vi "Read Peels.vi"(8 "error in (no error)":errorcluster, 11 "Banana in":refnum<class "Banana.lvclass">) -> (0 "error out":errorcluster, 2 "Peels":set{refnum<class "BananaPeel.lvclass">}(c389), 3 "Banana out":refnum<class "Banana.lvclass">)   [LabVIEW 2021, in "Bananas.lvlib" / "Banana.lvclass"]
uses:
  Banana.lvclass
  Banana.lvclass/Banana.ctl
  BananaPeel/BananaPeel.lvclass
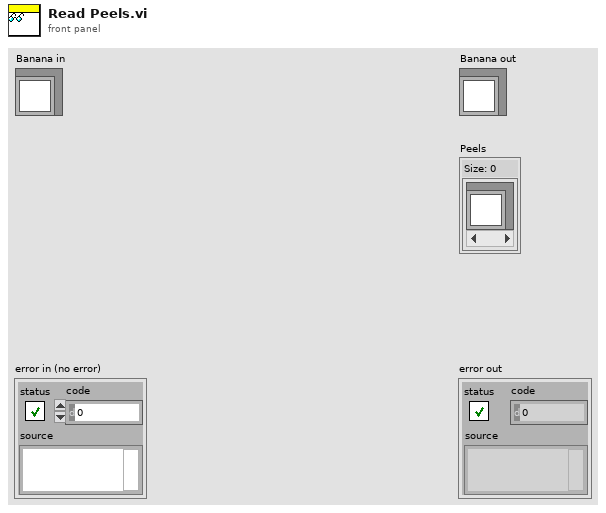
[diagram p1: front panel]
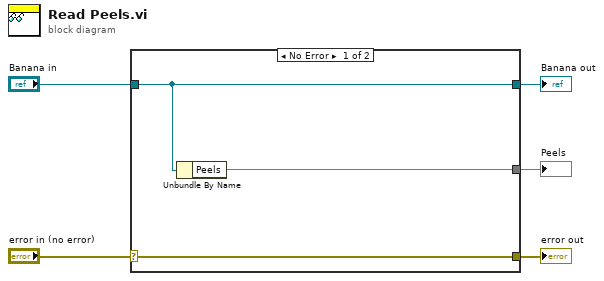
[diagram p0: block diagram]
diagram:
  n1 = case shown="No Error" "error in (no error)" {
    selector: "error in (no error)" -> [w8 w9]
    tunnel: [w8 w9] -> w4
    tunnel: [w7 w10] -> w2
    tunnel: "Banana in" -> [w7 w10]
    tunnel: [w6 _] -> w1
    frame No Error {
      n2 = Unbundle By Name(w7) -> ("Peels"=w6:set{refnum<class "BananaPeel.lvclass">})
    }
    frame Error {
    }
  }
  "error out" <- w4
  "Banana out" <- w2
  "Peels" <- w1
